vi "Injection Profile Generation for Testing.vi"() -> ()   [LabVIEW 2015]
panel:
  out "Current Sequence":dbl[][](graph)
  out "Voltage Sequence":dbl[][](graph)
  out "Voltage Input Graph":dbl[](graph)
  out "Current Input Graph":dbl[](graph)
  in  "Current Input":dbl[](array[numeric])=array[5015 elements]
  in  "Engine RPM":dbl=1000.0
  in  "SOI delay index array":dbl[](array[numeric])=[0.0, 0.0, 0.0, 0.0, 0.0, 0.0, 0.0, 0.0, 0.0, 0.0, 0.0, 0.0, 0.0, 0.0, 0.0, 0.0]
  in  "Voltage Input":dbl[](array[numeric])=array[5001 elements]
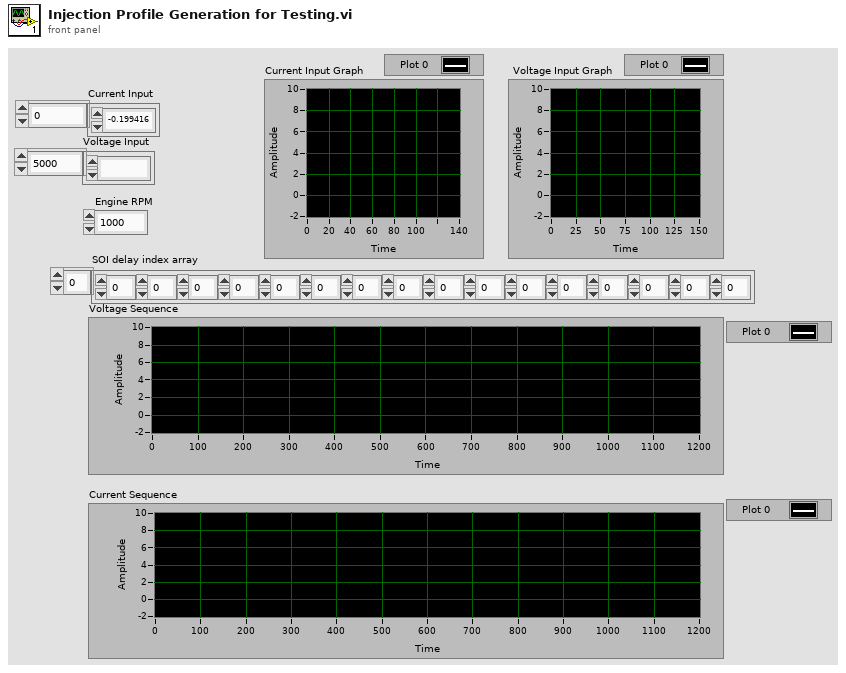
[diagram p1: front panel]
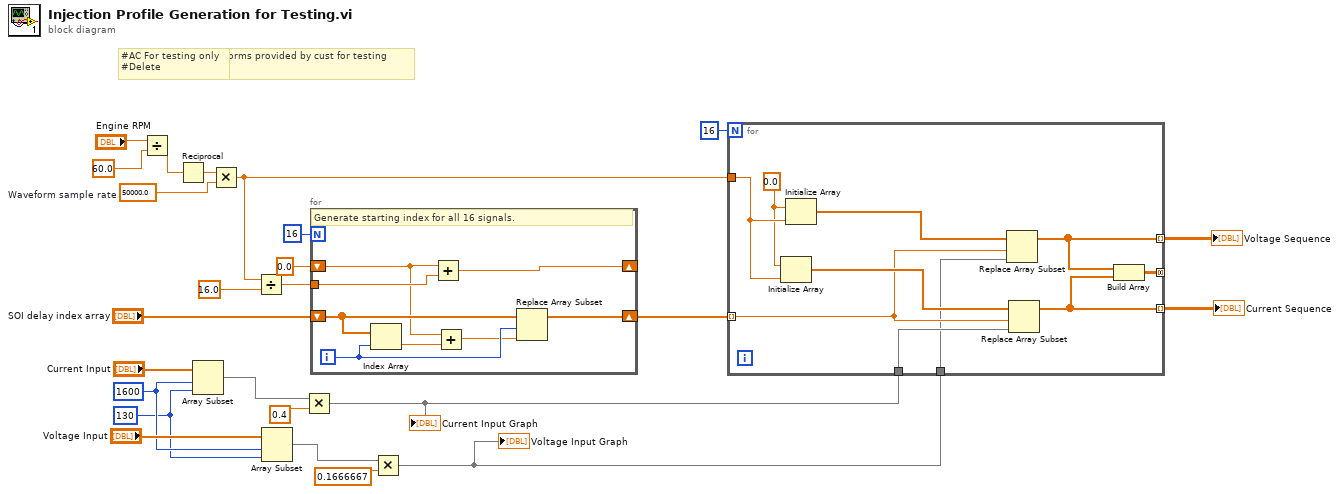
[diagram p0: block diagram]
diagram:
  w16 = 50000.0  # Waveform sample rate
  w2 = 130 ("length")
  w3 = 1600 ("index")
  # "#AC Generating waveforms provided by cust for testing\n#Remove"
  # "#AC For testing only\n#Delete"
  n1 = Divide(x="Engine RPM", y=60.0) -> (x/y=w14:dbl)
  n2 = Reciprocal(x=w14) -> (1/x=w15:dbl)
  n3 = Array Subset(array="Current Input", index=w3, length=w2) -> (w9:dbl[])
  n4 = Multiply(x=w15, y=w16) -> (x*y=w18:dbl)
  n5 = Divide(x=w18, y=16.0) -> (x/y=w21:dbl)
  n6 = Array Subset(array="Voltage Input", index=w3, length=w2) -> (w5:dbl[])
  n7 = Multiply(x=w9, y=0.4 ("Numeric")) -> (x*y=w24:dbl[])
  "Current Input Graph" <- w24
  n8 = for {
    N: 16 -> [_]
    shift-right: [w33] -> w23
    shift-left: "SOI delay index array" -> [w31]
    tunnel: w21 -> [w32]
    shift-right: [w28] -> _
    shift-left: 0.0 -> [w26]
    i -> [w30]
    # "Generate starting index for all 16 signals."
    n9 = Index Array(array=w31, index=w30) -> (element=w29:dbl)
    n10 = Add(x=w26, y=w32) -> (x+y=w28:dbl)
    n11 = Add(x=w26, y=w29) -> (x+y=w27:dbl)
    n12 = Replace Array Subset(array=w31, new element=w27, index=w30) -> (w33:dbl[])
  }
  n13 = Multiply(x=w5, y=0.1666667 ("Numeric")) -> (x*y=w1:dbl[])
  "Voltage Input Graph" <- w1
  n14 = for {
    N: 16 -> [_]
    tunnel: w18 -> [w42]
    tunnel: w23 -> [w39] mode=indexing
    tunnel: w24 -> [w38]
    tunnel: w1 -> [w37]
    tunnel: [w35] -> w8 mode=indexing
    tunnel: [w36] -> w7 mode=indexing
    tunnel: [w34] -> _ mode=concatenating
    w41 = 0.0 ("element")
    n15 = Initialize Array(w41, w42) -> (w40:dbl[])
    n16 = Initialize Array(w41, w42) -> (w43:dbl[])
    n17 = Replace Array Subset(array=w43, new element=w37, index=w39) -> (w36:dbl[])
    n18 = Replace Array Subset(array=w40, new element=w38, index=w39) -> (w35:dbl[])
    n19 = Build Array(w36, w35) -> (w34:dbl[][])
  }
  "Voltage Sequence" <- w7
  "Current Sequence" <- w8
